vi "MoveSegment.vi"(0 "Start X":dbl format="%#_13g", 1 "Start Y":dbl format="%#_13g", 2 "Start Z":dbl format="%#_13g", 3 "End X":dbl format="%#_13g", 4 "End Y":dbl format="%#_13g", 5 "End Z":dbl format="%#_13g", 6 "Number":i32) -> (14 "Comm1":string, 15 "Comm2":string, 16 "Comm":string[](array[string]))   [LabVIEW 2016]
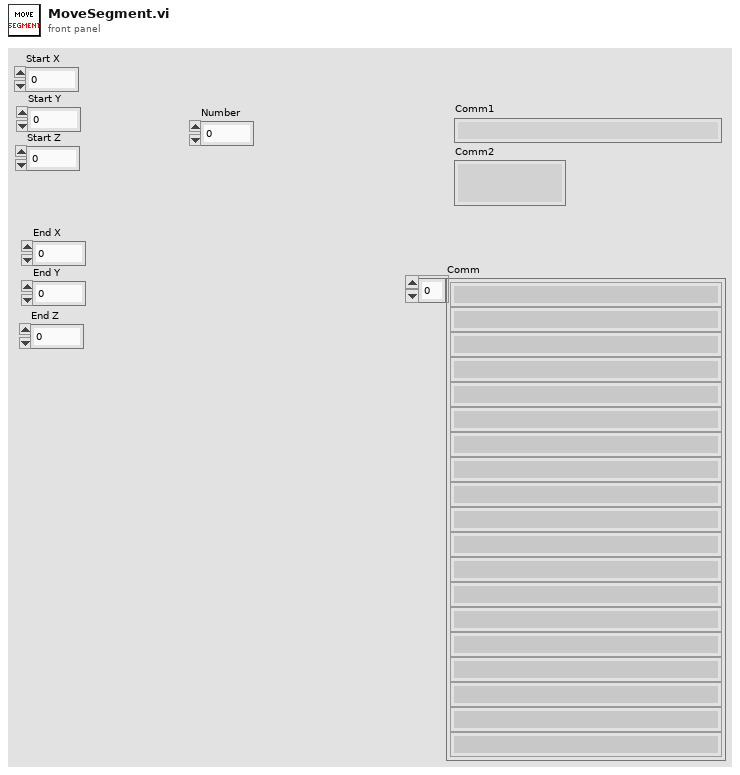
[diagram p1: front panel]
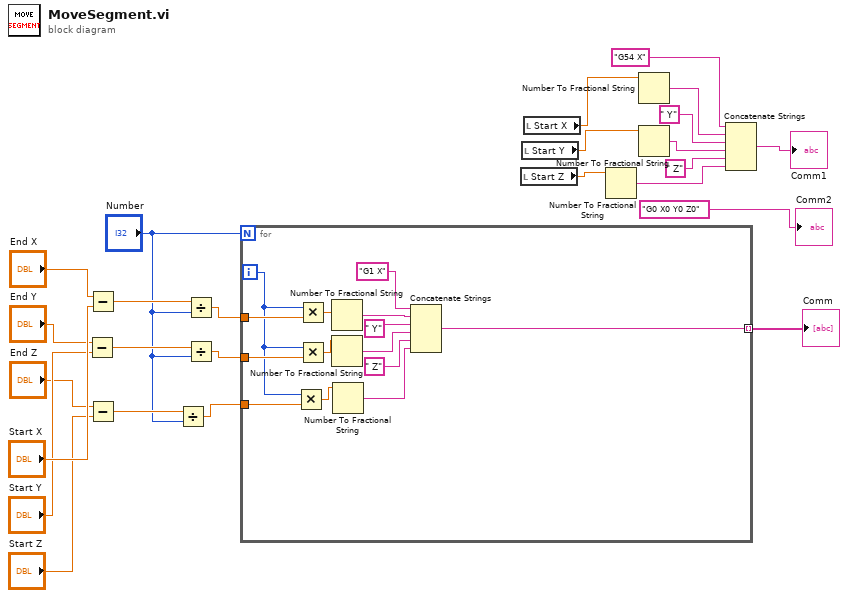
[diagram p0: block diagram]
diagram:
  n1 = Subtract(x="End Y", y="Start Y") -> (x-y=w18:dbl)
  n2 = Subtract(x="End X", y="Start X") -> (x-y=w19:dbl)
  n3 = Subtract(x="End Z", y="Start Z") -> (x-y=w17:dbl)
  n4 = Divide(x=w17, y="Number") -> (x/y=w13:dbl)
  n5 = Divide(x=w19, y="Number") -> (x/y=w15:dbl)
  n6 = Divide(x=w18, y="Number") -> (x/y=w14:dbl)
  n7 = for {
    N: "Number" -> [_]
    tunnel: w15 -> [w39]
    tunnel: w14 -> [w38]
    tunnel: w13 -> [w37]
    tunnel: [w28] -> w12 mode=indexing
    i -> [w36]
    n8 = Multiply(x=w36, y=w37) -> (x*y=w26:dbl)
    n9 = Multiply(x=w36, y=w39) -> (x*y=w34:dbl)
    n10 = Multiply(x=w36, y=w38) -> (x*y=w27:dbl)
    n11 = Number To Fractional String(number=w34) -> (F-format string=w33:string)  [unwired: 3 in]
    n12 = Number To Fractional String(number=w27) -> (F-format string=w31:string)  [unwired: 3 in]
    n13 = Number To Fractional String(number=w26) -> (F-format string=w29:string)  [unwired: 3 in]
    n14 = Concatenate Strings("G1 X", w33, " Y", w31, " Z", w29) -> (w28:string)
  }
  "Comm" <- w12
  n15 = local read "Start Z"() -> (w9:dbl)
  n16 = local read "Start Y"() -> (w10:dbl)
  n17 = local read "Start X"() -> (w11:dbl)
  n18 = Number To Fractional String(number=w9) -> (F-format string=w4:string)  [unwired: 3 in]
  n19 = Number To Fractional String(number=w11) -> (F-format string=w8:string)  [unwired: 3 in]
  n20 = Number To Fractional String(number=w10) -> (F-format string=w6:string)  [unwired: 3 in]
  n21 = Concatenate Strings("G54 X", w8, " Y", w6, " Z", w4) -> (→"Comm1":string)
  "Comm2" <- "G0 X0 Y0 Z0"
